vi "Override Error.vi"(10 "Error":errorcluster, 11 "qqqqq in":refnum<class "qqqqq.lvclass">) -> (3 "qqqqq out":refnum<class "qqqqq.lvclass">)   [LabVIEW 2021, in "jettl Tools.lvlib" / "qqqqq.lvlib" / "qqqqq.lvclass"]
uses:
  qqqqq.lvclass
  qqqqq.lvclass/qqqqq.ctl
  jettl/Queue/Queue.lvclass
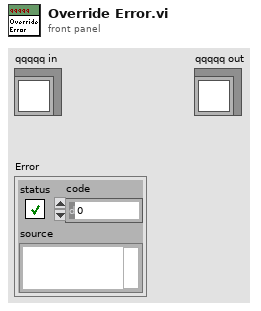
[diagram p1: front panel]
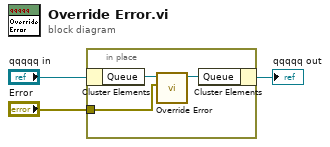
[diagram p0: block diagram]
diagram:
  n1 = in-place {
    in-place-border: "Error" -> [w4]
    n2 = in-place-cluster #1("qqqqq in") -> ("Queue"=w6:refnum<class "Queue.lvclass">)
    n3 = call-dynamic "Override Error.vi"("Error"=w4, "Override Error in"=w6) -> ("Override Error out"=w5:refnum<class "Queue.lvclass">)  [unwired: 9 in]
    n4 = in-place-cluster #1("Queue"=w5) -> (→"qqqqq out":refnum<class "qqqqq.lvclass">)
  }
